vi "Module Cleanup.vi"(8 "error in (no error)":errorcluster, 11 "Sequencing in":refnum<class "Sequencing.lvclass">) -> (0 "error out":errorcluster, 3 "Sequencing out":refnum<class "Sequencing.lvclass">)   [LabVIEW 2020, in "VolatusSeq.lvlib" / "Sequencing.lvclass"]
uses:
  Sequencing.lvclass
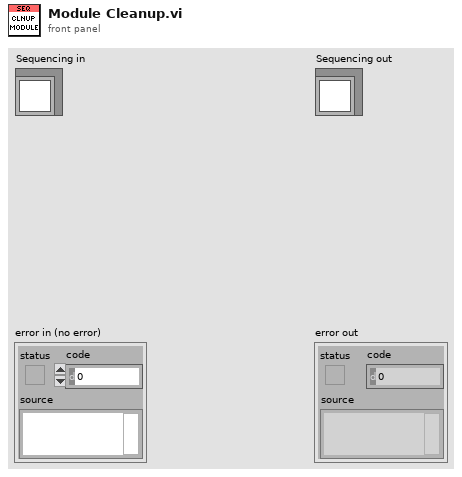
[diagram p1: front panel]
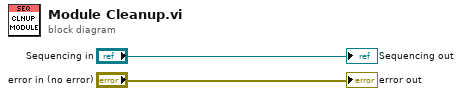
[diagram p0: block diagram]
diagram:
  "error out" <- "error in (no error)"
  "Sequencing out" <- "Sequencing in"
